vi "Create PUBREL Packet.vi"(5 "PUBREL in":refnum<class "PUBREL.lvclass">, 8 "error in (no error)":errorcluster, 9 "Packet ID":u16 format="%04x") -> (0 "error out":errorcluster, 2 "Bytes Stream":u8[](array[numeric]) format="%08b", 3 "PUBREL out":refnum<class "PUBREL.lvclass">)   [LabVIEW 2013, in "MQTT_Control_Packets.lvlib" / "PUBREL.lvclass"]
uses:
  PUBREL.lvclass
  ControlPacket/ControlPacket.lvclass/ControlPacket.ctl
  ControlPacket/ControlPacket.lvclass
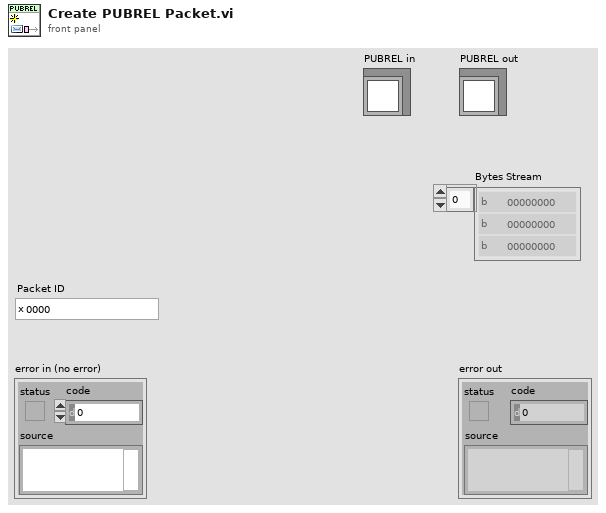
[diagram p1: front panel]
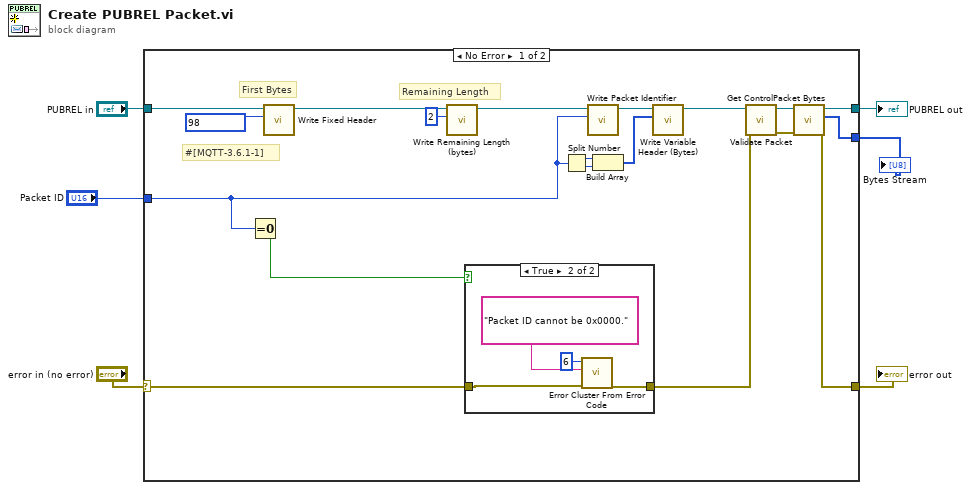
[diagram p0: block diagram]
diagram:
  n1 = case shown="No Error" "error in (no error)" {
    selector: "error in (no error)" -> [w14 w32]
    tunnel: [w9 w32] -> w3
    tunnel: [w7 w31] -> w2
    tunnel: "PUBREL in" -> [w25 w31]
    tunnel: "Packet ID" -> [w16 _]
    tunnel: [w11 _] -> w1
    frame No Error {
      # "#[MQTT-3.6.1-1]"
      # "Remaining Length"
      # "First Bytes"
      n2 = Equal To 0?(x=w16) -> (x = 0?=w15:bool)
      n3 = call "Write Fixed Header.vi"("Fixed Header"=u8 98, "ControlPacket in"=w25) -> ("ControlPacket out"=w24:refnum<class "PUBREL.lvclass">)  [unwired: 9 in]
      n4 = call "Write Remaining Length (bytes).vi"("Remaining Length (bytes)"=u32 2, "ControlPacket in"=w24) -> ("ControlPacket out"=w20:refnum<class "PUBREL.lvclass">)  [unwired: 9 in]
      n5 = case shown="True" w15 {
        tunnel: w14 -> [w26 w29]
        tunnel: [w26 w30] -> w12
        frame False {
        }
        frame True {
          n6 = call <vilib>:"Error Cluster From Error Code.vi"("error in (no error)"=w29, "error message (\"\")"="Packet ID cannot be 0x0000.", "error code (0)"=6) -> ("error out"=w30:errorcluster)  [unwired: 6 in]
        }
      }
      n7 = Split Number(x=w16) -> (hi(x)=w23:u8, lo(x)=w22:u8)
      n8 = call "Write Packet Identifier.vi"("Packet Identifier"=w16, "ControlPacket in"=w20) -> ("ControlPacket out"=w19:refnum<class "PUBREL.lvclass">)  [unwired: 9 in]
      n9 = Build Array(w23, w22) -> (w21:u8[])
      n10 = call "Write Variable Header (Bytes).vi"("Variable Header (Bytes)"=w21, "ControlPacket in"=w19) -> ("ControlPacket out"=w13:refnum<class "PUBREL.lvclass">)  [unwired: 9 in]
      n11 = call "Validate Packet.vi"("error in (no error)"=w12, "ControlPacket in"=w13) -> ("error out"=w10:errorcluster, "ControlPacket out"=w8:refnum<class "PUBREL.lvclass">)  [unwired: 8 in]
      n12 = call "Get ControlPacket Bytes.vi"("error in (no error)"=w10, "ControlPacket"=w8) -> ("error out"=w9:errorcluster, "Bytes Stream"=w11:u8[], "ControlPacket dup"=w7:refnum<class "PUBREL.lvclass">)  [unwired: 6 in, 1 out]
    }
    frame Error {
    }
  }
  "error out" <- w3
  "PUBREL out" <- w2
  "Bytes Stream" <- w1
